vi "Teardown.vi"(8 "error in (no error)":errorcluster, 11 "_Template in":refnum<class "_Template.lvclass">) -> (0 "error out":errorcluster)   [LabVIEW 2025, in "_Template.lvlib" / "_Template.lvclass"]
uses:
  _Template.lvclass
  _Template.lvclass/_Template.ctl
  _Shared/Project Stuff/Project Stuff.lvclass
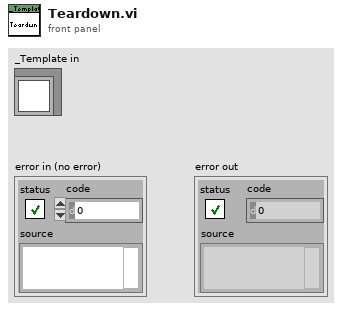
[diagram p1: front panel]
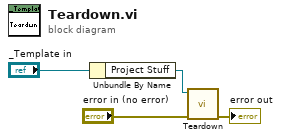
[diagram p0: block diagram]
diagram:
  n1 = Unbundle By Name("_Template in") -> ("Project Stuff"=w1:refnum<class "Project Stuff.lvclass">)
  n2 = call "Teardown.vi"("Error in"="error in (no error)", "Project Stuff in"=w1) -> ("Error out"=→"error out":errorcluster)  [unwired: 9 in]
